vi "Example Simple 2.vi"() -> ()   [LabVIEW 2010]
uses:
  C:/tf/play/labview/Tinkerforge.dll
  Tinkerforge.dll
panel:
  out "temperature (°C)":sgl
  out "humidity (%RH)":sgl
  in  "uid":string="Dkq"
  in  "port":i32=4223
  in  "host":string="localhost"
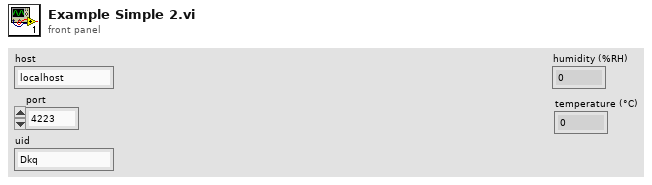
[diagram p1: front panel]
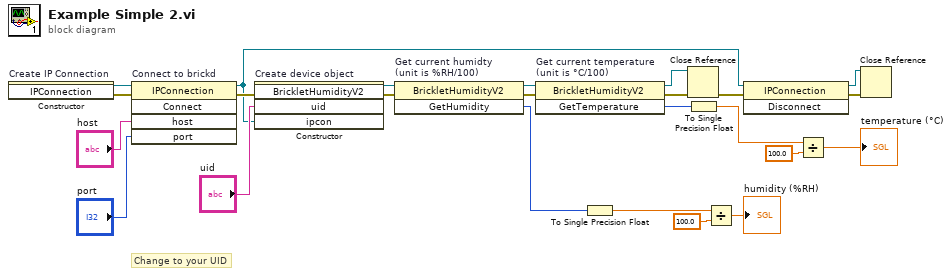
[diagram p0: block diagram]
diagram:
  # "Change to your UID"
  n1 = constructor on="Create IP Connection" class="IPConnection"() -> (reference out=w24:refnum<k24>, error out=w9:errorcluster)  [unwired: 3 in, 1 out]
  n2 = invoke on="Connect to brickd" class="IPConnection" method="Connect"(reference=w24, error in=w9, "host"="host", "port"="port") -> (reference out=w15:refnum<k24>, error out=w20:errorcluster)  [unwired: 1 in, 3 out]
  n3 = constructor on="Create device object" class="BrickletHumidityV2"(error in=w20, "uid"="uid", "ipcon"=w15) -> (reference out=w18:refnum<k24>, error out=w19:errorcluster)  [unwired: 2 in, 3 out]
  n4 = invoke on="Get current humidty\n(unit is %RH/100)" class="BrickletHumidityV2" method="GetHumidity"(reference=w18, error in=w19) -> (reference out=w2:refnum<k24>, error out=w4:errorcluster, "GetHumidity"=w13:i32)  [unwired: 1 in]
  n5 = invoke on="Get current temperature\n(unit is °C/100)" class="BrickletHumidityV2" method="GetTemperature"(reference=w2, error in=w4) -> (reference out=w1:refnum<k24>, error out=w3:errorcluster, "GetTemperature"=w8:i16)  [unwired: 1 in]
  n6 = To Single Precision Float(number=w13) -> (single precision float=w11:sgl)
  n7 = Close Reference(reference=w1, error in (no error)=w3) -> (error out=w17:errorcluster)
  n8 = To Single Precision Float(number=w8) -> (single precision float=w6:sgl)
  n9 = Divide(x=w11, y=sgl 100.0) -> (x/y=→"humidity (%RH)":sgl)
  n10 = invoke class="IPConnection" method="Disconnect"(reference=w15, error in=w17) -> (reference out=w14:refnum<k24>, error out=w16:errorcluster)  [unwired: 1 in, 1 out]
  n11 = Divide(x=w6, y=sgl 100.0) -> (x/y=→"temperature (°C)":sgl)
  n12 = Close Reference(reference=w14, error in (no error)=w16) -> ()  [unwired: 1 out]
